vi "Check ALL Iteration Metrics.vi"(0 "reference in":refnum<class "AdvSigProc.lvclass">, 5 "error in (no error)":errorcluster) -> (13 "Stop Iteration":bool, 14 "reference out":refnum<class "AdvSigProc.lvclass">, 19 "error out":errorcluster)   [LabVIEW 2022 SP3, in "AdvSigProc.lvclass"]
uses:
  AdvSigProc.lvclass
  API/GSwFormDSP_class/functions/TDF Parameters.ctl
  <vilib>/addons/Time Series Analysis/Correlation and Spectral Analysis.llb/TSA Cross-Correlation Function (Waveform).vi
  API/GSwFormDSP_class/GSwFormDSP.lvclass
  <vilib>/addons/_Advanced Signal Processing/NI_AdvSigProcTSA.lvlib
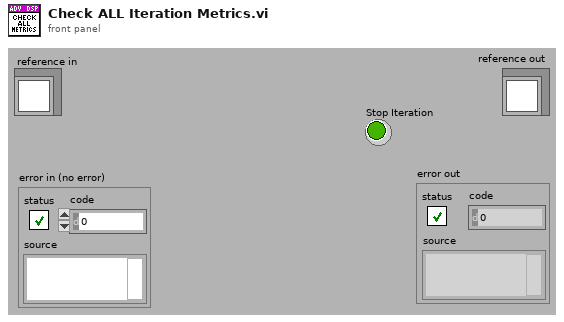
[diagram p1: front panel]
types:
  T1 = typedef "GSwFormDSP.lvclass/TDF Parameters.ctl" = cluster{"Filter":enum32{"Lowpass", "Highpass", "Bandpass", "Bandstop"}, "Type:":enum16{"Butterworth", "Chebyshev", "Inv Chebyshev", "Elliptic", "Bessel"}, "LP cutoff freq":dbl, "HP cutoff freq":dbl, "Order":i32, "passband ripple (dB)":dbl, "stopband attenuation (dB)":dbl, "Phaseless Filter":bool, "Include Fade IN and OUT":bool}
  T2 = typedef "AdvSigProc.lvclass/ObjectAttributesRef.ctl" = refnum<data-value>
  T3 = typedef "AdvSigProc.lvclass/ObjectAttributes.ctl" = cluster{"Time Data":cluster{"New Time Data Obj?":bool, "GSwFormDSP":refnum<class "GSwFormDSP.lvclass">}, "LMS Parameters":T4}
  T4 = typedef "AdvSigProc.lvclass/LMS.ctl" = cluster{"adaptive filter Ref":refnum<k20>, "Filtered Signals":refnum<class "GSwFormDSP.lvclass">, "Filter Coefs":dbl[], "Input Parameters":T5, "Iteration Metrics":T6[]}
  T5 = typedef "AdvSigProc.lvclass/LMS Input Parameters.ctl" = cluster{"Type":enum16{"Normalized LMS", "LMS", "FIR Sign LMS", "FIR Fast Block LMS", "RLS", "QR - RLS"}, "Filter Class":enum16{"Noise Cancelling (BGN Ref)", "Noise Cancelling (Speech Ref)"}, "Filter Length":i32, "µ Parameters":cluster{"Type":enum16{"User Input", "Auto µ"}, "step size":dbl}, "Iterations":cluster{"Current":i32, "Maximum":i32}}
  T6 = typedef "AdvSigProc.lvclass/Iteration Metrics.ctl" = cluster{"Name":string, "Max":dbl, "Min":dbl, "Values History":dbl[]}
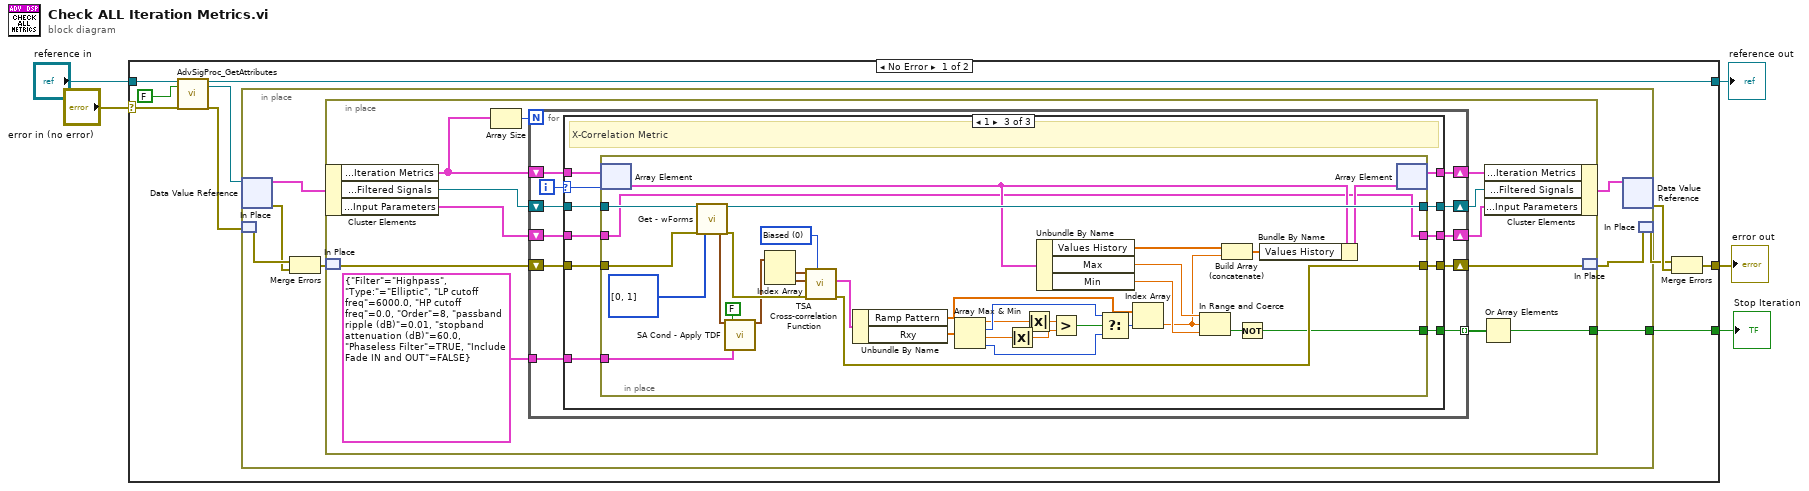
[diagram p0: block diagram]
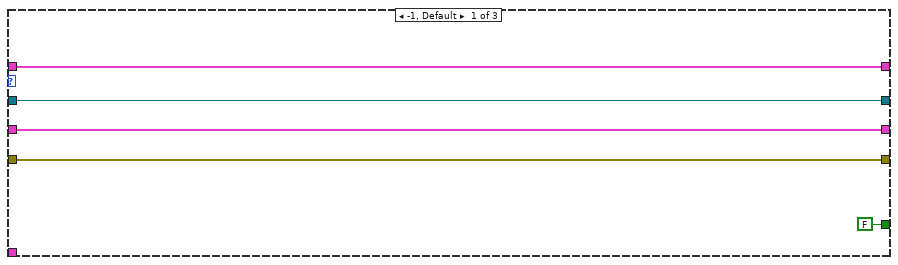
[diagram p2: hidden frame]
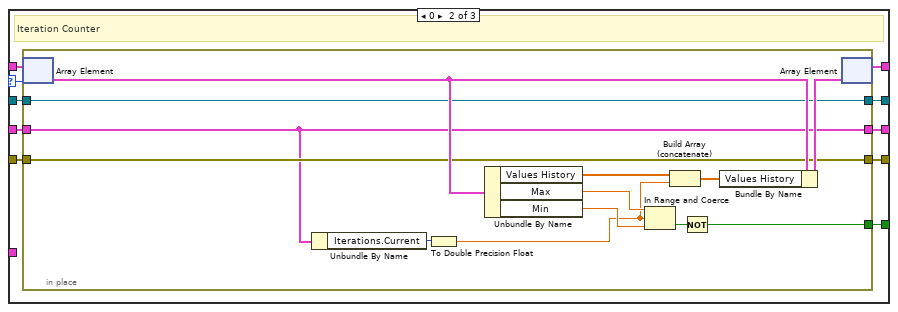
[diagram p3: hidden frame]
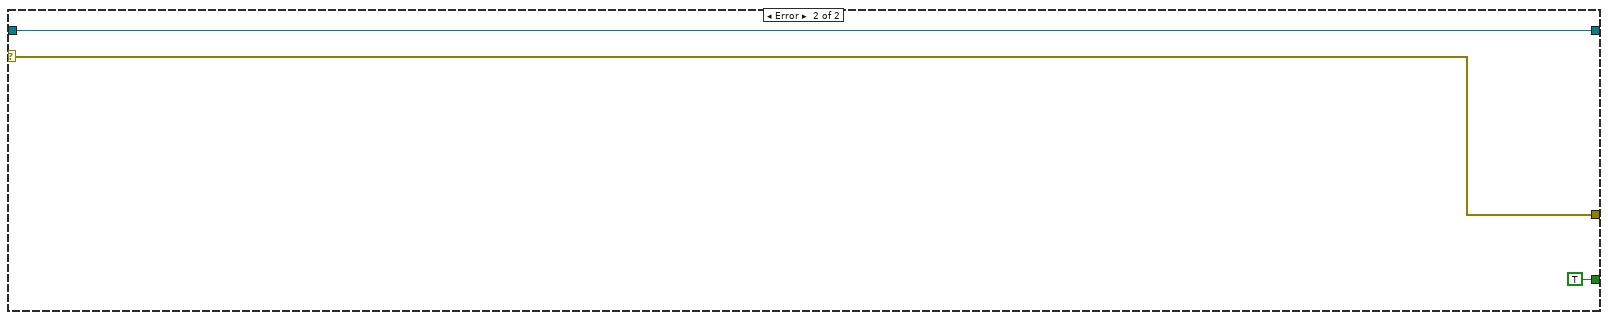
[diagram p4: hidden frame]
diagram:
  n1 = case shown="No Error" "error in (no error)" {
    selector: "error in (no error)" -> [w11 w121]
    tunnel: [w15 w121] -> w4
    tunnel: [w10 w120] -> w2
    tunnel: "reference in" -> [w13 w120]
    tunnel: [w6 TRUE] -> w1
    frame No Error {
      n2 = call "AdvSigProc_GetAttributes.vi"("reference in"=w13, "return data? (T)"=FALSE, "error in (no error)"=w11) -> ("reference out"=w10:refnum<class "AdvSigProc.lvclass">, "attributes ref"=w9:T2, "error out"=w8:errorcluster)  [unwired: 13 in, 1 out]
      n3 = in-place {
        in-place-border: [w16] -> w6
        n4 = in-place-dvr #1(w9) -> (w21:T3, w19:errorcluster)
        n5 = in-place-match #2(w8) -> (w20:errorcluster)
        n6 = Merge Errors(w20, w19) -> (w18:errorcluster)
        n7 = in-place {
          in-place-border: [w27] -> w16
          n8 = in-place-cluster #3(w21) -> ("LMS Parameters.Iteration Metrics"=w33:T6[], "LMS Parameters.Filtered Signals"=w31:refnum<class "GSwFormDSP.lvclass">, "LMS Parameters.Input Parameters"=w25:T5)
          n9 = in-place-match #4(w18) -> (w29:errorcluster)
          n10 = Array Size(array=w33) -> (size(s)=w34:i32)
          n11 = for {
            N: w34 -> [_]
            shift-right: [w44] -> w32
            shift-left: w33 -> [w45]
            shift-right: [w40] -> w30
            shift-left: w31 -> [w42]
            shift-right: [w39] -> w26
            shift-left: w29 -> [w41]
            tunnel: [w38] -> w28 mode=indexing
            shift-right: [w36] -> w24
            shift-left: w25 -> [w37]
            tunnel: T1 {"Filter"=enum."Highpass", "Type:"=enum."Elliptic", "LP cutoff freq"=6000.0, "HP cutoff freq"=0.0, "Order"=8, "passband ripple (dB)"=0.01, "stopband attenuation (dB)"=60.0, "Phaseless Filter"=TRUE, "Include Fade IN and OUT"=FALSE} ("TDF Parameters") -> [w35]
            i -> [w43]
            n12 = case shown="1" w43 {
              selector: w43 -> [_ w58 w82]
              tunnel: w45 -> [w50 w60 w84]
              tunnel: [w50 w59 w83] -> w44
              tunnel: [FALSE w53 w77] -> w38
              tunnel: w42 -> [w49 w57 w81]
              tunnel: w41 -> [w48 w56 w80]
              tunnel: [w49 w55 w79] -> w40
              tunnel: [w48 w54 w78] -> w39
              tunnel: w37 -> [w46 w52 w75]
              tunnel: [w46 w51 w76] -> w36
              tunnel: w35 -> [_ _ w74]
              frame -1, Default {
              }
              frame 0 {
                # "Iteration Counter"
                n13 = in-place {
                  in-place-border: w57 -> [w65]
                  in-place-border: w56 -> [w64]
                  in-place-border: [w65] -> w55
                  in-place-border: [w64] -> w54
                  in-place-border: [w70] -> w53
                  in-place-border: w52 -> [w61]
                  in-place-border: [w61] -> w51
                  n14 = in-place-array #5(w60, w58) -> (w69:T6)
                  n15 = Unbundle By Name(w61) -> ("Iterations.Current"=w63:i32)
                  n16 = To Double Precision Float(number=w63) -> (double precision float=w62:dbl)
                  n17 = Unbundle By Name(w69) -> ("Values History"=w67:dbl[], "Max"=w72:dbl, "Min"=w73:dbl)
                  n18 = In Range and Coerce(upper limit=w72, x=w62, lower limit=w73) -> (In Range?=w71:bool)  [unwired: 1 out]
                  n19 = Build Array (concatenate)(w67, w62) -> (w66:dbl[])
                  n20 = Not(x=w71) -> (.not. x?=w70:bool)
                  n21 = Bundle By Name(cluster=w69, "Values History"=w66) -> (w68:T6)
                  n22 = in-place-array #5(w68) -> (w59:T6[])  [unwired: 1 out]
                }
              }
              frame 1 {
                # "X-Correlation Metric"
                n23 = in-place {
                  in-place-border: w81 -> [w118]
                  in-place-border: w80 -> [w117]
                  in-place-border: [w115] -> w79
                  in-place-border: [w100] -> w78
                  in-place-border: [w96] -> w77
                  in-place-border: [w89] -> w76
                  in-place-border: w75 -> [w89]
                  in-place-border: w74 -> [w85]
                  w102 = u16 0 items=["Biased", "Unbiased"] ("weighting")
                  n24 = in-place-array #6(w84, w82) -> (w95:T6)
                  n25 = call-dynamic "Get - wForms.vi"("reference in"=w118, "error in (no error)"=w117, "Indexes (Empty = ALL)"=i32[] [0, 1]) -> ("wForms"=w88:waveform(dbl)[], "reference out"=w115:refnum<class "GSwFormDSP.lvclass">, "error out"=w101:errorcluster)  [unwired: 13 in, 1 out]
                  n26 = call "SA Cond - Apply TDF.vi"("Signals IN"=w88, "Anotate Signal Name"=FALSE, "TDF Parameters"=w85) -> ("Signals OUT"=w86:waveform(dbl)[])  [unwired: 16 in]
                  n27 = Index Array(array=w86) -> (element #1=w90:waveform(dbl), element #2=w103:waveform(dbl))  [unwired: 2 in]
                  n28 = call-poly <vilib>:"TSA Cross-correlation Function.vi"("weighting"=w102, "error in (no error)"=w101, "Yt"=w103, "Xt"=w90) -> ("error out"=w100:errorcluster, "correlogram"=w114:cluster{"Ramp Pattern":dbl[], "Rxy":dbl[]})  [unwired: 1 in, 5 out]
                  n29 = Unbundle By Name(w114) -> ("Ramp Pattern"=w107:dbl[], "Rxy"=w113:dbl[])
                  n30 = Array Max & Min(array=w113) -> (max value=w105:dbl, max index (indices)=w110:i32, min value=w104:dbl, min index (indices)=w109:i32)
                  n31 = Absolute Value(x=w104) -> (abs(x)=w111:dbl)
                  n32 = Absolute Value(x=w105) -> (abs(x)=w112:dbl)
                  n33 = Unbundle By Name(w95) -> ("Values History"=w93:dbl[], "Max"=w98:dbl, "Min"=w99:dbl)
                  n34 = Greater?(x=w112, y=w111) -> (0:w106:bool)
                  n35 = Select(t=w110, s=w106, f=w109) -> (s? t:f=w108:i32)
                  n36 = Index Array(array=w107, index=w108) -> (element=w92:dbl)
                  n37 = In Range and Coerce(upper limit=w98, x=w92, lower limit=w99) -> (In Range?=w97:bool)  [unwired: 1 out]
                  n38 = Build Array (concatenate)(w93, w92) -> (w91:dbl[])
                  n39 = Not(x=w97) -> (.not. x?=w96:bool)
                  n40 = Bundle By Name(cluster=w95, "Values History"=w91) -> (w94:T6)
                  n41 = in-place-array #6(w94) -> (w83:T6[])  [unwired: 1 out]
                }
              }
            }
          }
          n42 = Or Array Elements(Boolean array=w28) -> (logical OR=w27:bool)
          n43 = in-place-cluster #3("LMS Parameters.Iteration Metrics"=w32, "LMS Parameters.Filtered Signals"=w30, "LMS Parameters.Input Parameters"=w24) -> (w22:T3)
          n44 = in-place-match #4(w26) -> (w17:errorcluster)
        }
        n45 = in-place-dvr #1(w22) -> (w14:errorcluster)  [unwired: 1 out]
        n46 = in-place-match #2(w17) -> (w7:errorcluster)
      }
      n47 = Merge Errors(w7, w14) -> (w15:errorcluster)
    }
    frame Error {
    }
  }
  "error out" <- w4
  "reference out" <- w2
  "Stop Iteration" <- w1
